vi "VAT_valve_get_software_version.vi"(0 "VAT Valve COM port":refnum<visa-resource-name>, 11 "error in (no error)":errorcluster) -> (4 "VAT Valve COM port out":refnum<visa-resource-name>, 13 "Software Version":dbl format="%#_6f", 15 "error out":errorcluster)   [LabVIEW 2019]
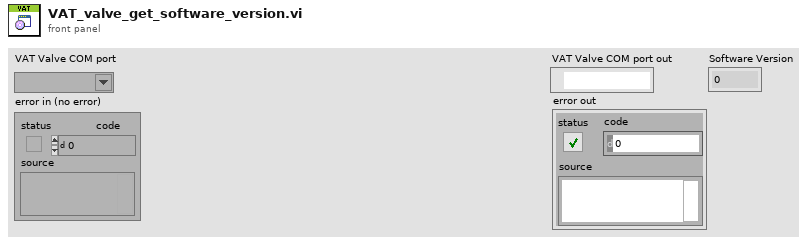
[diagram p1: front panel]
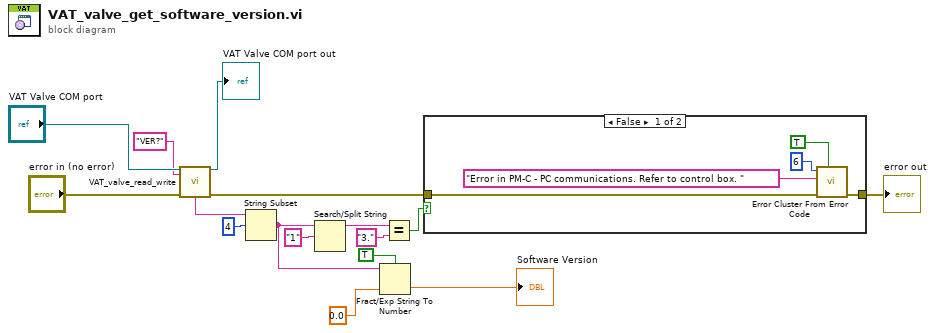
[diagram p0: block diagram]
diagram:
  n1 = call "VAT_valve_read_write.vi"("VAT Valve COM port"="VAT Valve COM port", "Write String"="VER?", "error in (no error)"="error in (no error)") -> ("VAT Valve COM port out"=→"VAT Valve COM port out":refnum<visa-resource-name>, "Read String"=w7:string, "error out"=w10:errorcluster)  [unwired: 10 in]
  n2 = String Subset(string=w7, offset (0)=4) -> (substring=w1:string)  [unwired: 1 in]
  n3 = Search/Split String(string=w1, search string/char (-)="1") -> (substring before match=w5:string)  [unwired: 1 in, 2 out]
  n4 = Fract/Exp String To Number(use system decimal point (T)=TRUE, string=w1, default (0 dbl)=0.0) -> (number=→"Software Version":dbl)  [unwired: 1 in, 1 out]
  n5 = Equal?(x=w5, y="3.") -> (x = y?=w13:bool)
  n6 = case shown="False" w13 {
    tunnel: [w18 w22] -> w12
    tunnel: w10 -> [w17 w22]
    frame False {
      n7 = call <vilib>:"Error Cluster From Error Code.vi"("show call chain? (False)"=TRUE, "error in (no error)"=w17, "error message (\"\")"="Error in PM-C - PC communications. Refer to control box. " ("error message (\"\")"), "error code (0)"=6) -> ("error out"=w18:errorcluster)  [unwired: 5 in]
    }
    frame True {
    }
  }
  "error out" <- w12
